vi "Do.vi"(8 "error in (no error)":errorcluster, 10 "Actor in":refnum<class "Actor.lvclass">, 11 "Handle Activate Menu On Tree Item Msg":refnum<class "Handle Activate Menu On Tree Item Msg.lvclass">) -> (0 "error out":errorcluster, 2 "Actor out":refnum<class "Actor.lvclass">)   [LabVIEW 2020, in "File Explorer.lvlib" / "Handle Activate Menu On Tree Item Msg.lvclass"]
doc: "This VI delivers the message to the actor by calling the appropriate method(s) on the actor."
uses:
  <vilib>/gpm_packages/@cs/file-explorer-extension/Source/File Explorer/File Explorer Messages/Handle Activate Menu On Tree Item Msg/Handle Activate Menu On Tree Item Msg.lvclass
  <vilib>/ActorFramework/Actor/Actor.lvclass
  <vilib>/gpm_packages/@cs/file-explorer-extension/Source/File Explorer/File Explorer/File Explorer.lvclass
  C:/Program Files/National Instruments/LabVIEW 2020/vi.lib/ActorFramework/Actor/Actor.lvclass
  <vilib>/gpm_packages/@cs/file-explorer-extension/Source/File Explorer/File Explorer Messages/Handle Activate Menu On Tree Item Msg/Handle Activate Menu On Tree Item Msg.lvclass/Handle Activate Menu On Tree Item Msg.ctl
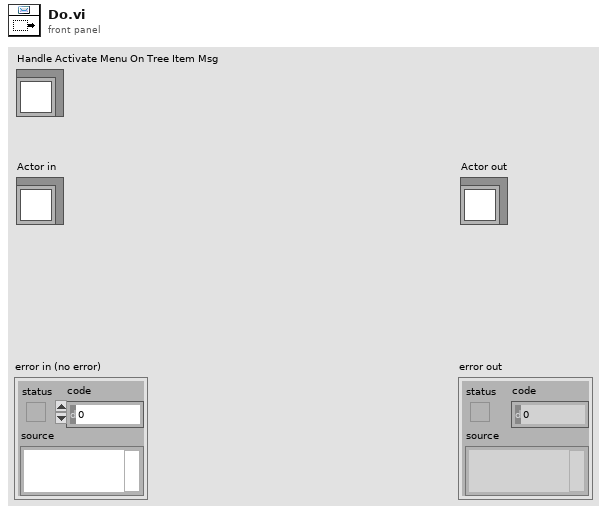
[diagram p1: front panel]
types:
  T1 = typedef "LVPoint32TypeDef.ctl" = cluster{"Horizontal":i32, "Vertical":i32}
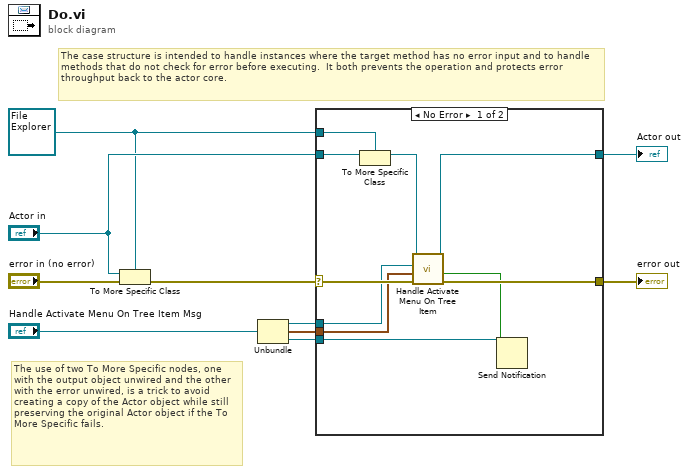
[diagram p0: block diagram]
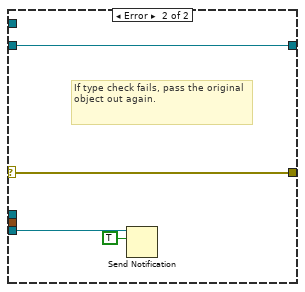
[diagram p2: hidden frame]
diagram:
  w4 = refnum<class "File Explorer.lvclass"> refnum ("Actor in")
  # "The use of two To More Specific nodes, one with the output object unwired and the other with the error unwired, is a trick to avoid creating a copy of the Actor object while still preserving the original Actor object if the To More Specific fails."
  # "The case structure is intended to handle instances where the target method has no error input and to handle methods that do not check for error before executing.  It both prevents the operation and protects error throughput back to the actor core."
  n1 = To More Specific Class(target class=w4, reference="Actor in", error in="error in (no error)") -> (error out=w8:errorcluster)  [unwired: 1 out]
  n2 = Unbundle("Handle Activate Menu On Tree Item Msg") -> (w3:refnum<k9>, w2:T1, w1:refnum<notifier>)
  n3 = case shown="No Error" w8 {
    selector: w8 -> [w18 w24]
    tunnel: [w20 w24] -> w7
    tunnel: [w19 w23] -> w6
    tunnel: "Actor in" -> [w17 w23]
    tunnel: w4 -> [w16 _]
    tunnel: w3 -> [w14 _]
    tunnel: w2 -> [w13 _]
    tunnel: w1 -> [w12 w22]
    frame No Error {
      n4 = To More Specific Class(target class=w16, reference=w17) -> (specific class reference=w15:refnum<class "File Explorer.lvclass">)  [unwired: 1 in, 1 out]
      n5 = call-dynamic "Handle Activate Menu On Tree Item.vi"("error in (no error)"=w18, "Coords"=w13, "MenuRef"=w14, "File Explorer in"=w15) -> ("error out"=w20:errorcluster, "Discard?"=w11:bool, "File Explorer out"=w19:refnum<class "File Explorer.lvclass">)  [unwired: 5 in]
      n6 = Send Notification(notification=w11, notifier=w12) -> ()  [unwired: 1 in, 2 out]
    }
    frame Error {
      # "If type check fails, pass the original object out again."
      n7 = Send Notification(notification=TRUE, notifier=w22) -> ()  [unwired: 1 in, 2 out]
    }
  }
  "error out" <- w7
  "Actor out" <- w6
